vi "LSMcontroller_v59_PIzstage.vi"() -> ()   [LabVIEW 2015] (continued)
                n3606 = Unbundle By Name(w327) -> ("AOtab"=w308:dbl, "Repeats"=w326:dbl, "Cycles"=w325:dbl, "Start amplitude (V)"=w324:dbl, "Baseline (V)"=w323:dbl, "Step size (V)"=w322:dbl, "DC (%)"=w321:dbl, "Sampling frequency (Hz)"=w320:dbl, "Period (ms)"=w319:dbl, "Offset (V)"=w318:dbl, "Amplitude (V)"=w317:dbl, "Frequency"=w316:dbl, "Tri Repeats"=w315:dbl, "phase shift (ms)"=w314:dbl, "Pulses"=w313:dbl, "Tri phase"=w309:dbl, "padding value"=w305:dbl, "Matlab wave file"=w306:path)
                n3607 = To Unsigned Long Integer(number=w308) -> (unsigned 32bit integer=w307:u32)
                n3608 = local write "Build analog waveform tabs"(w307) -> ()
                n3609 = local write "Matlab waveform path"(w306) -> ()
                n3610 = local write "phase shift (ms)"(w314) -> ()
                n3611 = local write "Repeats"(w326) -> ()
                n3612 = local write "Cycles"(w325) -> ()
                n3613 = local write "Amplitude (V)"(w317) -> ()
                n3614 = local write "Matlab padding value"(w305) -> ()
                n3615 = local write "Tri padding value"(w305) -> ()
                n3616 = local write "Start amplitude (V)"(w324) -> ()
                n3617 = local write "Tri Phase (s)"(w309) -> ()
                n3618 = local write "Period (ms)"(w319) -> ()
                n3619 = local write "Tri Repeats"(w315) -> ()
                n3620 = local write "Offset (V)"(w318) -> ()
                n3621 = local write "Frequency"(w316) -> ()
                n3622 = local write "Pulses"(w313) -> ()
                n3623 = local write "padding value"(w305) -> ()
                n3624 = local write "Sampling rate \ncurrent wf"(w320) -> ()
                n3625 = local write "Baseline (V)"(w323) -> ()
                n3626 = local write "Step size (V)"(w322) -> ()
                n3627 = local write "DC (%)"(w321) -> ()
              }
              frame True {
              }
            }
          }
          event "Rem AO wave": Value Change {
            n3628 = event-data() -> ("NewVal"=w328:bool)  [unwired: 1 in, 5 out]
            n3629 = case shown="True" w328 {
              frame False {
              }
              frame True {
                n3630 = stacked-sequence {
                  seq-local: [_ _ w434 _ _ _ _] -> [_ _ _ _ w454 w457 _]
                  frame #0 {
                    n3631 = local read "Measurement"() -> (w329:T4)
                    n3632 = case shown="\"X-Y-t movie\", Default" w329 {
                      frame "X-Y-t movie", Default {
                        n3633 = local read "avpp"() -> (w350:i32)
                        n3634 = local read "Angle ref"() -> (w349:dbl)
                        n3635 = local read "ROI Type"() -> (w348:u16)
                        n3636 = local read "xpixels ref"() -> (w345:i32)
                        n3637 = local read "Vx-min ref"() -> (w344:dbl)
                        n3638 = local read "Vx-max ref"() -> (w343:dbl)
                        n3639 = local read "ypixels ref"() -> (w341:i32)
                        n3640 = local read "Vy-min ref"() -> (w342:dbl)
                        n3641 = local read "Vy-max ref"() -> (w338:dbl)
                        n3642 = local read "Sampling rate"() -> (w332:dbl)
                        n3643 = local read "finite samples"() -> (w333:bool)
                        n3644 = local read "continuous"() -> (w336:bool)
                        n3645 = local read "wavdet"() -> (w337:bool)
                        n3646 = local read "# of frames"() -> (w335:i32)
                        n3647 = local read "maxbufferAI"() -> (w334:i32)
                        n3648 = local read "Override AI buffer"() -> (w330:bool)
                        n3649 = call "2pparameters.vi"("command"="get") -> ("params out"=w347:T11)  [unwired: 1 in]
                        n3650 = Bundle By Name(cluster=w347, "type"="X-Y-t movie", "avpp"=w350, "Angle Img"=w349, "Xpixels Img"=w345, "Vx-min Img"=w344, "VX-max Img"=w343, "Ypixels Img"=w341, "Vy-min Img"=w342, "Vy-max Img"=w338, "srate"=w332, "srate Img"=w332, "finite"=w333, "cont"=w336, "wavdet"=w337, "measpoints"=w335, "maxbufferAI"=w334, "Drawing Mode"=w348, "Vz-reset"=0.0, "AIoverride"=w330) -> (w339:T11)
                        n3651 = call "2pparameters.vi"("Params in"=w339, "command"="set") -> ()  [unwired: 1 out]
                      }
                      frame "X-Y-Z stack" {
                        n3652 = call "2pparameters.vi"("command"="get") -> ("params out"=w354:T11)  [unwired: 1 in]
                        n3653 = Bundle By Name(cluster=w354, "type"="X-Y-Z stack") -> (w352:T11)
                        n3654 = call "2pparameters.vi"("Params in"=w352, "command"="set") -> ()  [unwired: 1 out]
                      }
                      frame "Lifetime (scan)" {
                        n3655 = call "2pparameters.vi"("command"="get") -> ("params out"=w359:T11)  [unwired: 1 in]
                        n3656 = Bundle By Name(cluster=w359, "type"="Lifetime (scan)") -> (w357:T11)
                        n3657 = call "2pparameters.vi"("Params in"=w357, "command"="set") -> ()  [unwired: 1 out]
                      }
                      frame "Lifetime (contour)" {
                        n3658 = local read "Vy-min draw"() -> (w369:dbl)
                        n3659 = local read "Vy-max draw"() -> (w368:dbl)
                        n3660 = local read "Vx-min draw"() -> (w371:dbl)
                        n3661 = local read "Vx-max draw"() -> (w370:dbl)
                        n3662 = local read "xpixels ref"() -> (w367:i32)
                        n3663 = local read "ypixels ref"() -> (w366:i32)
                        n3664 = local read "ROI Type"() -> (w365:u16)
                        n3665 = local read "srateAODOtt"() -> (w376:dbl)
                        n3666 = local read "# of frames"() -> (w381:i32)
                        n3667 = local read "refreshtime"() -> (w373:dbl)
                        n3668 = local read "Pel"() -> (w364:dbl)
                        n3669 = local read "bin"() -> (w379:dbl)
                        n3670 = local read "Override AI buffer"() -> (w362:bool)
                        n3671 = local read "finite samples"() -> (w388:bool)
                        n3672 = local read "srateAODOtt"() -> (w375:dbl)
                        n3673 = local read "srateAODOtt"() -> (w382:dbl)
                        n3674 = local read "continuous"() -> (w387:bool)
                        n3675 = local read "Angle ref"() -> (w372:dbl)
                        n3676 = local read "wavdet"() -> (w389:bool)
                        n3677 = local read "Vx-ref"() -> (w384:dbl)
                        n3678 = local read "Vy-ref"() -> (w386:dbl)
                        n3679 = local read "avpp"() -> (w385:i32)
                        n3680 = call "tt_timeandsamples.vi"("bin"=w379, "refreshtime"=w373, "srateAODOtt"=w376, "tot#ofsamples"=w381) -> ("refreshrate"=w377:dbl, "refreshbuffer"=w378:i32, "timetracecycles"=w383:i32)  [unwired: 5 in]
                        n3681 = local read "bin"() -> (w380:dbl)
                        n3682 = call "2pparameters.vi"("command"="get") -> ("params out"=w392:T11)  [unwired: 1 in]
                        n3683 = Bundle By Name(cluster=w392, "Drawing Mode"=w365, "measpoints"=w381, "tt_cycles"=w383, "refreshbuffer"=w378, "refreshrate"=w377, "Vx-ref"=w384, "Vy-ref"=w386, "srate"=w375, "finite"=w388, "cont"=w387, "wavdet"=w389, "avpp"=w385, "srateAODO"=w382, "bufferAI"=w378, "bin"=w380, "Angle Img"=w372, "Vxminref"=w371, "Vxmaxref"=w370, "Vyminref"=w369, "Vymaxref"=w368, "Xpixels Img"=w367, "Ypixels Img"=w366, "Pel"=w364, "Vz-reset"=0.0, "AIoverride"=w362, "type"="Lifetime (contour)") -> (w390:T11)
                        n3684 = Reciprocal(x=w377) -> (1/x=w374:dbl)
                        n3685 = local write "refreshtime"(w374) -> ()
                        n3686 = call "2pparameters.vi"("Params in"=w390, "command"="set") -> ()  [unwired: 1 out]
                      }
                      frame "X-Y-Z-t movie" {
                      }
                      frame "linescan" {
                      }
                      frame "Timetrace" {
                        n3687 = local read "Vy-min draw"() -> (w402:dbl)
                        n3688 = local read "Vy-max draw"() -> (w401:dbl)
                        n3689 = local read "Vx-min draw"() -> (w404:dbl)
                        n3690 = local read "Vx-max draw"() -> (w403:dbl)
                        n3691 = local read "xpixels ref"() -> (w400:i32)
                        n3692 = local read "ypixels ref"() -> (w399:i32)
                        n3693 = local read "ROI Type"() -> (w398:u16)
                        n3694 = local read "srateAODOtt"() -> (w409:dbl)
                        n3695 = local read "# of frames"() -> (w414:i32)
                        n3696 = local read "refreshtime"() -> (w406:dbl)
                        n3697 = local read "Pel"() -> (w397:dbl)
                        n3698 = local read "bin"() -> (w412:dbl)
                        n3699 = local read "Override AI buffer"() -> (w395:bool)
                        n3700 = local read "finite samples"() -> (w421:bool)
                        n3701 = local read "srateAODOtt"() -> (w408:dbl)
                        n3702 = local read "srateAODOtt"() -> (w415:dbl)
                        n3703 = local read "continuous"() -> (w420:bool)
                        n3704 = local read "Angle ref"() -> (w405:dbl)
                        n3705 = local read "wavdet"() -> (w422:bool)
                        n3706 = local read "Vx-ref"() -> (w417:dbl)
                        n3707 = local read "Vy-ref"() -> (w419:dbl)
                        n3708 = local read "avpp"() -> (w418:i32)
                        n3709 = call "tt_timeandsamples.vi"("bin"=w412, "refreshtime"=w406, "srateAODOtt"=w409, "tot#ofsamples"=w414) -> ("refreshrate"=w410:dbl, "refreshbuffer"=w411:i32, "timetracecycles"=w416:i32)  [unwired: 5 in]
                        n3710 = local read "bin"() -> (w413:dbl)
                        n3711 = call "2pparameters.vi"("command"="get") -> ("params out"=w425:T11)  [unwired: 1 in]
                        n3712 = Bundle By Name(cluster=w425, "Drawing Mode"=w398, "measpoints"=w414, "tt_cycles"=w416, "refreshbuffer"=w411, "refreshrate"=w410, "Vx-ref"=w417, "Vy-ref"=w419, "srate"=w408, "finite"=w421, "cont"=w420, "wavdet"=w422, "avpp"=w418, "srateAODO"=w415, "bufferAI"=w411, "bin"=w413, "Angle Img"=w405, "Vxminref"=w404, "Vxmaxref"=w403, "Vyminref"=w402, "Vymaxref"=w401, "Xpixels Img"=w400, "Ypixels Img"=w399, "Pel"=w397, "Vz-reset"=0.0, "AIoverride"=w395, "type"="Timetrace") -> (w423:T11)
                        n3713 = Reciprocal(x=w410) -> (1/x=w407:dbl)
                        n3714 = local write "refreshtime"(w407) -> ()
                        n3715 = call "2pparameters.vi"("Params in"=w423, "command"="set") -> ()  [unwired: 1 out]
                      }
                      frame "Lifetime (point)" {
                      }
                    }
                  }
                  frame #1 {
                    w428 = FALSE ("wavdet")
                    n3716 = call "2pparameters.vi"("command"="get") -> ("params out"=w432:T11)  [unwired: 1 in]
                    n3717 = Bundle By Name(cluster=w432, "finite"=w428, "cont"=w428, "wavdet"=TRUE) -> (w429:T11)
                    n3718 = call "2pparameters.vi"("Params in"=w429, "command"="set") -> ()  [unwired: 1 out]
                  }
                  frame #2 {
                    # "remove channel from numbers array"
                    n3719 = local read "AO channels"() -> (w439:u32)
                    n3720 = call "2pparameters.vi"("command"="get") -> ("params out"=w437:T11)  [unwired: 1 in]
                    n3721 = in-place {
                      in-place-border: w439 -> [w445]
                      in-place-border: [w442] -> w440
                      in-place-border: [w441] -> w434
                      n3722 = in-place-cluster #50(w437) -> ("aAO"=w444:u32[])
                      n3723 = call "remove channel from active arrayv2.vi"("line array in"=w444, "line to remove"=w445) -> ("line array out"=w443:u32[], "removal"=w442:bool, "index"=w441:i32)
                      n3724 = in-place-cluster #50("aAO"=w443) -> (w435:T11)
                    }
                    n3725 = local write "remAO"(w440) -> ()
                    n3726 = call "2pparameters.vi"("Params in"=w435, "command"="set") -> ()  [unwired: 1 out]
                  }
                  frame #3 {
                    n3727 = local read "remAO"() -> (w446:bool)
                    n3728 = case shown="True" w446 {
                      frame False {
                      }
                      frame True {
                        n3729 = call "Used AO lines.vi"() -> ("used AO names"=w450:string[], "used AO lines"=w452:tag[])  [unwired: 2 in]
                        n3730 = control-ref of="Analog Lines Plot"() -> (w451:refnum<vi>)
                        n3731 = control-ref of="Digital Lines Plot"() -> (w449:refnum<vi>)
                        n3732 = call "Used DO lines.vi"() -> ("used DO names"=w448:string[], "used DO lines"=w447:tag[])  [unwired: 2 in]
                        n3733 = local write "Analog Used Lines"(w452) -> ()
                        n3734 = local write "Analog Used Names"(w450) -> ()
                        n3735 = local write "Digital Used Lines"(w447) -> ()
                        n3736 = local write "Digital Used Names"(w448) -> ()
                        n3737 = call "prepDOWaveplot.vi"("DigitalGraph in"=w449, "used DO names"=w448) -> ()  [unwired: 1 in]
                        n3738 = call "prepAOWaveplot.vi"("WaveformGraph in"=w451, "Analog Used Names"=w450) -> ()  [unwired: 1 in]
                      }
                    }
                  }
                  frame #4 {
                    n3739 = local read "remAO"() -> (w453:bool)
                    n3740 = case shown="True" w453 {
                      tunnel: w454 -> [_ w455]
                      frame False {
                      }
                      frame True {
                        n3741 = call "waveformparamsv2.vi"("command"="rem AO", "index"=w455) -> ()  [unwired: 3 in, 3 out]
                      }
                    }
                  }
                  frame #5 {
                    n3742 = local read "remAO"() -> (w458:bool)
                    n3743 = case shown="True" w458 {
                      tunnel: w457 -> [_ w477]
                      frame False {
                      }
                      frame True {
                        n3744 = local read "Meastab"() -> (w462:enum32{"X-Y Image", "Linescan", "Timetrace"})
                        n3745 = property on="refwf" class="Ring (strict)"() -> ("RingText.Text"=w465:string)  [unwired: 2 in, 2 out]
                        n3746 = case shown="\"Timetrace\"" w462 {
                          tunnel: [w478 w479] -> w461
                          frame "X-Y Image", Default {
                            n3747 = local read "Sampling rate"() -> (w478:dbl)
                          }
                          frame "Timetrace" {
                            n3748 = local read "srateAODOtt"() -> (w479:dbl)
                          }
                        }
                        n3749 = call "waveformsAObuffer.vi"("command"="get") -> ("AO wf out"=w474:waveform(dbl)[])  [unwired: 1 in]
                        n3750 = call "waveformsDObuffer.vi"("command"="get") -> ("DO wf out"=w471:digitalwaveform[])  [unwired: 1 in]
                        n3751 = Delete From Array(array=w474, length=1, index=w477) -> (array with subset deleted=w466:waveform(dbl)[])  [unwired: 1 out]
                        n3752 = call "correctwaveformsizetemp.vi"("new sampling frequency (Hz)"=w461, "start"=FALSE, "reference waveforms to"=w465, "Analog waveforms in"=w466, "stop"=FALSE, "Digital waveforms in"=w471) -> ("analog wf out"=w469:waveform(dbl)[], "Digital wf out"=w467:digitalwaveform[], "measpoints"=w463:i32)
                        n3753 = local write "Analog Lines Plot"(w469) -> ()
                        n3754 = call "GetNumCamFramesv2.vi"("Digital Waveform Graph"=w467) -> ("Numeric"=w468:i32)  [unwired: 10 in]
                        n3755 = local write "Digital Lines Plot"(w467) -> ()
                        n3756 = call "waveformsAObuffer.vi"("AO wf in"=w469, "command"="set") -> ()  [unwired: 1 out]
                        n3757 = call "waveformsDObuffer.vi"("DO wf in"=w467, "command"="set") -> ()  [unwired: 1 out]
                        n3758 = local read "wavdet"() -> (w464:bool)
                        n3759 = local write "Total Camera Frames"(w468) -> ()
                        n3760 = case shown="True" w464 {
                          tunnel: w463 -> [_ w480]
                          frame False {
                          }
                          frame True {
                            n3761 = local write "# of frames"(w480) -> ()
                          }
                        }
                      }
                    }
                  }
                  frame #6 {
                    w481 = FALSE ("remAO")
                    n3762 = local read "finite samples"() -> (w482:bool)
                    n3763 = local read "continuous"() -> (w483:bool)
                    n3764 = local read "wavdet"() -> (w484:bool)
                    n3765 = call "2pparameters.vi"("command"="get") -> ("params out"=w487:T11)  [unwired: 1 in]
                    n3766 = Bundle By Name(cluster=w487, "finite"=w482, "cont"=w483, "wavdet"=w484) -> (w485:T11)
                    n3767 = local write "remAO"(w481) -> ()
                    n3768 = property on="Rem AO wave" class="Bool (strict)"("Val(Sgnl)"=w481) -> ()  [unwired: 2 in, 2 out]
                    n3769 = call "2pparameters.vi"("Params in"=w485, "command"="set") -> ()  [unwired: 1 out]
                  }
                }
              }
            }
          }
          event "Add DO wave": Value Change {
            n3770 = event-data() -> ("NewVal"=w489:bool)  [unwired: 1 in, 5 out]
            n3771 = case shown="True" w489 {
              frame False {
              }
              frame True {
                n3772 = stacked-sequence {
                  seq-local: [_ _ _ _ _ w649 _ _] -> [_ _ _ _ _ _ w664 _]
                  frame #0 {
                    n3773 = local read "Measurement"() -> (w490:T4)
                    n3774 = case shown="\"X-Y-t movie\", Default" w490 {
                      frame "X-Y-t movie", Default {
                        n3775 = local read "avpp"() -> (w511:i32)
                        n3776 = local read "Angle ref"() -> (w510:dbl)
                        n3777 = local read "ROI Type"() -> (w509:u16)
                        n3778 = local read "xpixels ref"() -> (w506:i32)
                        n3779 = local read "Vx-min ref"() -> (w505:dbl)
                        n3780 = local read "Vx-max ref"() -> (w504:dbl)
                        n3781 = local read "ypixels ref"() -> (w502:i32)
                        n3782 = local read "Vy-min ref"() -> (w503:dbl)
                        n3783 = local read "Vy-max ref"() -> (w499:dbl)
                        n3784 = local read "Sampling rate"() -> (w493:dbl)
                        n3785 = local read "finite samples"() -> (w494:bool)
                        n3786 = local read "continuous"() -> (w497:bool)
                        n3787 = local read "wavdet"() -> (w498:bool)
                        n3788 = local read "# of frames"() -> (w496:i32)
                        n3789 = local read "maxbufferAI"() -> (w495:i32)
                        n3790 = local read "Override AI buffer"() -> (w491:bool)
                        n3791 = call "2pparameters.vi"("command"="get") -> ("params out"=w508:T11)  [unwired: 1 in]
                        n3792 = Bundle By Name(cluster=w508, "type"="X-Y-t movie", "avpp"=w511, "Angle Img"=w510, "Xpixels Img"=w506, "Vx-min Img"=w505, "VX-max Img"=w504, "Ypixels Img"=w502, "Vy-min Img"=w503, "Vy-max Img"=w499, "srate"=w493, "srate Img"=w493, "finite"=w494, "cont"=w497, "wavdet"=w498, "measpoints"=w496, "maxbufferAI"=w495, "Drawing Mode"=w509, "Vz-reset"=0.0, "AIoverride"=w491) -> (w500:T11)
                        n3793 = call "2pparameters.vi"("Params in"=w500, "command"="set") -> ()  [unwired: 1 out]
                      }
                      frame "X-Y-Z stack" {
                        n3794 = call "2pparameters.vi"("command"="get") -> ("params out"=w515:T11)  [unwired: 1 in]
                        n3795 = Bundle By Name(cluster=w515, "type"="X-Y-Z stack") -> (w513:T11)
                        n3796 = call "2pparameters.vi"("Params in"=w513, "command"="set") -> ()  [unwired: 1 out]
                      }
                      frame "Lifetime (scan)" {
                        n3797 = call "2pparameters.vi"("command"="get") -> ("params out"=w520:T11)  [unwired: 1 in]
                        n3798 = Bundle By Name(cluster=w520, "type"="Lifetime (scan)") -> (w518:T11)
                        n3799 = call "2pparameters.vi"("Params in"=w518, "command"="set") -> ()  [unwired: 1 out]
                      }
                      frame "Lifetime (contour)" {
                        n3800 = local read "Vy-min draw"() -> (w530:dbl)
                        n3801 = local read "Vy-max draw"() -> (w529:dbl)
                        n3802 = local read "Vx-min draw"() -> (w532:dbl)
                        n3803 = local read "Vx-max draw"() -> (w531:dbl)
                        n3804 = local read "xpixels ref"() -> (w528:i32)
                        n3805 = local read "ypixels ref"() -> (w527:i32)
                        n3806 = local read "ROI Type"() -> (w526:u16)
                        n3807 = local read "srateAODOtt"() -> (w537:dbl)
                        n3808 = local read "# of frames"() -> (w542:i32)
                        n3809 = local read "refreshtime"() -> (w534:dbl)
                        n3810 = local read "Pel"() -> (w525:dbl)
                        n3811 = local read "bin"() -> (w540:dbl)
                        n3812 = local read "Override AI buffer"() -> (w523:bool)
                        n3813 = local read "finite samples"() -> (w549:bool)
                        n3814 = local read "srateAODOtt"() -> (w536:dbl)
                        n3815 = local read "srateAODOtt"() -> (w543:dbl)
                        n3816 = local read "continuous"() -> (w548:bool)
                        n3817 = local read "Angle ref"() -> (w533:dbl)
                        n3818 = local read "wavdet"() -> (w550:bool)
                        n3819 = local read "Vx-ref"() -> (w545:dbl)
                        n3820 = local read "Vy-ref"() -> (w547:dbl)
                        n3821 = local read "avpp"() -> (w546:i32)
                        n3822 = call "tt_timeandsamples.vi"("bin"=w540, "refreshtime"=w534, "srateAODOtt"=w537, "tot#ofsamples"=w542) -> ("refreshrate"=w538:dbl, "refreshbuffer"=w539:i32, "timetracecycles"=w544:i32)  [unwired: 5 in]
                        n3823 = local read "bin"() -> (w541:dbl)
                        n3824 = call "2pparameters.vi"("command"="get") -> ("params out"=w553:T11)  [unwired: 1 in]
                        n3825 = Bundle By Name(cluster=w553, "Drawing Mode"=w526, "measpoints"=w542, "tt_cycles"=w544, "refreshbuffer"=w539, "refreshrate"=w538, "Vx-ref"=w545, "Vy-ref"=w547, "srate"=w536, "finite"=w549, "cont"=w548, "wavdet"=w550, "avpp"=w546, "srateAODO"=w543, "bufferAI"=w539, "bin"=w541, "Angle Img"=w533, "Vxminref"=w532, "Vxmaxref"=w531, "Vyminref"=w530, "Vymaxref"=w529, "Xpixels Img"=w528, "Ypixels Img"=w527, "Pel"=w525, "Vz-reset"=0.0, "AIoverride"=w523, "type"="Lifetime (contour)") -> (w551:T11)
                        n3826 = Reciprocal(x=w538) -> (1/x=w535:dbl)
                        n3827 = local write "refreshtime"(w535) -> ()
                        n3828 = call "2pparameters.vi"("Params in"=w551, "command"="set") -> ()  [unwired: 1 out]
                      }
                      frame "X-Y-Z-t movie" {
                      }
                      frame "linescan" {
                      }
                      frame "Timetrace" {
                        n3829 = local read "Vy-min draw"() -> (w563:dbl)
                        n3830 = local read "Vy-max draw"() -> (w562:dbl)
                        n3831 = local read "Vx-min draw"() -> (w565:dbl)
                        n3832 = local read "Vx-max draw"() -> (w564:dbl)
                        n3833 = local read "xpixels ref"() -> (w561:i32)
                        n3834 = local read "ypixels ref"() -> (w560:i32)
                        n3835 = local read "ROI Type"() -> (w559:u16)
                        n3836 = local read "srateAODOtt"() -> (w570:dbl)
                        n3837 = local read "# of frames"() -> (w575:i32)
                        n3838 = local read "refreshtime"() -> (w567:dbl)
                        n3839 = local read "Pel"() -> (w558:dbl)
                        n3840 = local read "bin"() -> (w573:dbl)
                        n3841 = local read "Override AI buffer"() -> (w556:bool)
                        n3842 = local read "finite samples"() -> (w582:bool)
                        n3843 = local read "srateAODOtt"() -> (w569:dbl)
                        n3844 = local read "srateAODOtt"() -> (w576:dbl)
                        n3845 = local read "continuous"() -> (w581:bool)
                        n3846 = local read "Angle ref"() -> (w566:dbl)
                        n3847 = local read "wavdet"() -> (w583:bool)
                        n3848 = local read "Vx-ref"() -> (w578:dbl)
                        n3849 = local read "Vy-ref"() -> (w580:dbl)
                        n3850 = local read "avpp"() -> (w579:i32)
                        n3851 = call "tt_timeandsamples.vi"("bin"=w573, "refreshtime"=w567, "srateAODOtt"=w570, "tot#ofsamples"=w575) -> ("refreshrate"=w571:dbl, "refreshbuffer"=w572:i32, "timetracecycles"=w577:i32)  [unwired: 5 in]
                        n3852 = local read "bin"() -> (w574:dbl)
                        n3853 = call "2pparameters.vi"("command"="get") -> ("params out"=w586:T11)  [unwired: 1 in]
                        n3854 = Bundle By Name(cluster=w586, "Drawing Mode"=w559, "measpoints"=w575, "tt_cycles"=w577, "refreshbuffer"=w572, "refreshrate"=w571, "Vx-ref"=w578, "Vy-ref"=w580, "srate"=w569, "finite"=w582, "cont"=w581, "wavdet"=w583, "avpp"=w579, "srateAODO"=w576, "bufferAI"=w572, "bin"=w574, "Angle Img"=w566, "Vxminref"=w565, "Vxmaxref"=w564, "Vyminref"=w563, "Vymaxref"=w562, "Xpixels Img"=w561, "Ypixels Img"=w560, "Pel"=w558, "Vz-reset"=0.0, "AIoverride"=w556, "type"="Timetrace") -> (w584:T11)
                        n3855 = Reciprocal(x=w571) -> (1/x=w568:dbl)
                        n3856 = local write "refreshtime"(w568) -> ()
                        n3857 = call "2pparameters.vi"("Params in"=w584, "command"="set") -> ()  [unwired: 1 out]
                      }
                      frame "Lifetime (point)" {
                      }
                    }
                  }
                  frame #1 {
                    w589 = FALSE ("wavdet")
                    n3858 = call "2pparameters.vi"("command"="get") -> ("params out"=w593:T11)  [unwired: 1 in]
                    n3859 = Bundle By Name(cluster=w593, "finite"=w589, "cont"=w589, "wavdet"=TRUE) -> (w590:T11)
                    n3860 = call "2pparameters.vi"("Params in"=w590, "command"="set") -> ()  [unwired: 1 out]
                  }
                  frame #2 {
                    n3861 = local read "DO channels"() -> (w600:u16)
                    n3862 = call "2pparameters.vi"("command"="get") -> ("params out"=w598:T11)  [unwired: 1 in]
                    n3863 = in-place {
                      in-place-border: w600 -> [w604]
                      in-place-border: [w601] -> w595
                      n3864 = in-place-cluster #51(w598) -> ("aDO"=w603:u32[])
                      n3865 = call "add channel to active arrayv2.vi"("line array in"=w603, "line to add"=w604) -> ("line array out"=w602:u32[], "addition"=w601:bool)  [unwired: 1 out]
                      n3866 = in-place-cluster #51("aDO"=w602) -> (w596:T11)
                    }
                    n3867 = local write "addDO"(w595) -> ()
                    n3868 = call "2pparameters.vi"("Params in"=w596, "command"="set") -> ()  [unwired: 1 out]
                  }
                  frame #3 {
                    n3869 = local read "addDO"() -> (w605:bool)
                    n3870 = case shown="True" w605 {
                      frame False {
                      }
                      frame True {
                        n3871 = call "Used AO lines.vi"() -> ("used AO names"=w609:string[], "used AO lines"=w611:tag[])  [unwired: 2 in]
                        n3872 = control-ref of="Analog Lines Plot"() -> (w610:refnum<vi>)
                        n3873 = control-ref of="Digital Lines Plot"() -> (w608:refnum<vi>)
                        n3874 = call "Used DO lines.vi"() -> ("used DO names"=w607:string[], "used DO lines"=w606:tag[])  [unwired: 2 in]
                        n3875 = local write "Analog Used Lines"(w611) -> ()
                        n3876 = local write "Analog Used Names"(w609) -> ()
                        n3877 = local write "Digital Used Lines"(w606) -> ()
                        n3878 = local write "Digital Used Names"(w607) -> ()
                        n3879 = call "prepDOWaveplot.vi"("DigitalGraph in"=w608, "used DO names"=w607) -> ()  [unwired: 1 in]
                        n3880 = call "prepAOWaveplot.vi"("WaveformGraph in"=w610, "Analog Used Names"=w609) -> ()  [unwired: 1 in]
                      }
                    }
                  }
                  frame #4 {
                    n3881 = local read "addDO"() -> (w612:bool)
                    n3882 = case shown="True" w612 {
                      frame False {
                      }
                      frame True {
                        n3883 = local read "Build digital waveform tabs"() -> (w613:enum32{"Simple", "Matlab"})
                        n3884 = case shown="\"Matlab\"" w613 {
                          frame "Simple", Default {
                            n3885 = local read "Meastab"() -> (w615:enum32{"X-Y Image", "Linescan", "Timetrace"})
                            n3886 = call "waveformparamsv2.vi"("command"="get") -> ("Params out"=w629:T15)  [unwired: 4 in, 2 out]
                            n3887 = case shown="\"Timetrace\"" w615 {
                              tunnel: [w631 w632] -> w614
                              frame "X-Y Image", Default {
                                n3888 = local read "Sampling rate"() -> (w631:dbl)
                              }
                              frame "Timetrace" {
                                n3889 = local read "srateAODOtt"() -> (w632:dbl)
                              }
                            }
                            n3890 = Unbundle By Name(w629) -> ("DO parameters"=w627:T18)
                            n3891 = local read "Digital padding value"() -> (w618:dbl)
                            n3892 = local read "Digital time offset (s)"() -> (w619:dbl)
                            n3893 = local read "Digital phase (s)"() -> (w621:dbl)
                            n3894 = local read "Digital Freq (Hz)"() -> (w620:dbl)
                            n3895 = local read "Digital DC (%)"() -> (w622:dbl)
                            n3896 = Index Array(array=w627, index=0) -> (element=w626:T19)
                            n3897 = Bundle By Name(cluster=w626, "Digital DC (%)"=w622, "Digital phase"=w621, "Digital Freq (Hz)"=w620, "Sampling frequency (Hz)"=w614, "Digital time offset (s)"=w619, "padding value"=w618, "matlab wave file"=path "", "DOtab"=0.0) -> (w624:T19)
                            n3898 = Build Array(w624) -> (w623:T18)
                            n3899 = call "waveformparamsv2.vi"("command"="add DO", "add DO"=w623) -> ()  [unwired: 3 in, 3 out]
                          }
                          frame "Matlab" {
                            w636 = 0.0 ("DOtab")
                            n3900 = local read "Meastab"() -> (w634:enum32{"X-Y Image", "Linescan", "Timetrace"})
                            n3901 = call "waveformparamsv2.vi"("command"="get") -> ("Params out"=w645:T15)  [unwired: 4 in, 2 out]
                            n3902 = case shown="\"Timetrace\"" w634 {
                              tunnel: [w647 w648] -> w633
                              frame "X-Y Image", Default {
                                n3903 = local read "Sampling rate"() -> (w647:dbl)
                              }
                              frame "Timetrace" {
                                n3904 = local read "srateAODOtt"() -> (w648:dbl)
                              }
                            }
                            n3905 = Unbundle By Name(w645) -> ("DO parameters"=w643:T18)
                            n3906 = local read "Matlab waveform path DO"() -> (w635:path)
                            n3907 = local read "Matlab padding value DO"() -> (w638:dbl)
                            n3908 = Index Array(array=w643, index=0) -> (element=w642:T19)
                            n3909 = Bundle By Name(cluster=w642, "Digital DC (%)"=w636, "Digital phase"=w636, "Digital Freq (Hz)"=w636, "Sampling frequency (Hz)"=w633, "Digital time offset (s)"=w636, "padding value"=w638, "matlab wave file"=w635, "DOtab"=1.0) -> (w640:T19)
                            n3910 = Build Array(w640) -> (w639:T18)
                            n3911 = call "waveformparamsv2.vi"("command"="add DO", "add DO"=w639) -> ()  [unwired: 3 in, 3 out]
                          }
                        }
                      }
                    }
                  }
                  frame #5 {
                    n3912 = local read "addDO"() -> (w650:bool)
                    n3913 = case shown="True" w650 {
                      tunnel: [_ w651] -> w649
                      frame False {
                      }
                      frame True {
                        n3914 = property on="refwf" class="Ring (strict)"() -> ("RingText.Text"=w656:string)  [unwired: 2 in, 2 out]
                        n3915 = call "waveformsDObuffer.vi"("command"="get") -> ("DO wf out"=w655:digitalwaveform[])  [unwired: 1 in]
                        n3916 = call "waveformsAObuffer.vi"("command"="get") -> ("AO wf out"=w653:waveform(dbl)[])  [unwired: 1 in]
                        n3917 = call "referfencesize.vi"("Digital waveforms in"=w655, "Analog waveforms in"=w653, "reference waveforms to"=w656) -> ("number of samples"=w651:i32)  [unwired: 2 in]
                      }
                    }
                  }
                  frame #6 {
                    n3918 = local read "Build digital waveform tabs"() -> (w667:enum32{"Simple", "Matlab"})
                    n3919 = call "waveformparamsv2.vi"("command"="get last DO") -> ("last DO"=w666:T19)  [unwired: 4 in, 2 out]
                    n3920 = local read "Meastab"() -> (w660:enum32{"X-Y Image", "Linescan", "Timetrace"})
                    n3921 = call "waveformsDObuffer.vi"("command"="get") -> ("DO wf out"=w665:digitalwaveform[])  [unwired: 1 in]
                    n3922 = case shown="\"Simple\", Default" w667 {
                      tunnel: w666 -> [w684 w686]
                      tunnel: w664 -> [w683 _]
                      tunnel: [w682 w685] -> w663
                      frame "Simple", Default {
                        n3923 = call "simple digital from wf params.vi"("waveform params"=w684, "number of samples"=w683) -> ("digital waveform"=w682:digitalwaveform)
                      }
                      frame "Matlab" {
                        n3924 = call "matlabDOwffromparam.vi"("waveform params"=w686) -> ("digital waveform"=w685:digitalwaveform)
                      }
                    }
                    n3925 = property on="refwf" class="Ring (strict)"() -> ("RingText.Text"=w670:string)  [unwired: 2 in, 2 out]
                    n3926 = case shown="\"Timetrace\"" w660 {
                      tunnel: [w679 w680] -> w659
                      frame "X-Y Image", Default {
                        n3927 = local read "Sampling rate"() -> (w679:dbl)
                      }
                      frame "Timetrace" {
                        n3928 = local read "srateAODOtt"() -> (w680:dbl)
                      }
                    }
                    n3929 = call "waveformsAObuffer.vi"("command"="get") -> ("AO wf out"=w678:waveform(dbl)[])  [unwired: 1 in]
                    n3930 = Build Array (concatenate)(w665, w663) -> (w669:digitalwaveform[])
                    n3931 = call "correctwaveformsizetemp.vi"("new sampling frequency (Hz)"=w659, "start"=FALSE, "reference waveforms to"=w670, "Analog waveforms in"=w678, "stop"=FALSE, "Digital waveforms in"=w669) -> ("analog wf out"=w673:waveform(dbl)[], "Digital wf out"=w671:digitalwaveform[], "measpoints"=w661:i32)
                    n3932 = local write "Analog Lines Plot"(w673) -> ()
                    n3933 = call "GetNumCamFramesv2.vi"("Digital Waveform Graph"=w671) -> ("Numeric"=w672:i32)  [unwired: 10 in]
                    n3934 = local write "Digital Lines Plot"(w671) -> ()
                    n3935 = call "waveformsAObuffer.vi"("AO wf in"=w673, "command"="set") -> ()  [unwired: 1 out]
                    n3936 = call "waveformsDObuffer.vi"("DO wf in"=w671, "command"="set") -> ()  [unwired: 1 out]
                    n3937 = local write "Total Camera Frames"(w672) -> ()
                    n3938 = local read "wavdet"() -> (w662:bool)
                    n3939 = case shown="True" w662 {
                      tunnel: w661 -> [_ w681]
                      frame False {
                      }
                      frame True {
                        n3940 = local write "# of frames"(w681) -> ()
                      }
                    }
                  }
                  frame #7 {
                    w687 = FALSE ("addAO")
                    n3941 = local read "finite samples"() -> (w688:bool)
                    n3942 = local read "continuous"() -> (w689:bool)
                    n3943 = local read "wavdet"() -> (w690:bool)
                    n3944 = call "2pparameters.vi"("command"="get") -> ("params out"=w693:T11)  [unwired: 1 in]
                    n3945 = Bundle By Name(cluster=w693, "finite"=w688, "cont"=w689, "wavdet"=w690) -> (w691:T11)
                    n3946 = call "2pparameters.vi"("Params in"=w691, "command"="set") -> ()  [unwired: 1 out]
                    n3947 = local write "addDO"(w687) -> ()
                    n3948 = property on="Add DO wave" class="Bool (strict)"("Val(Sgnl)"=w687) -> ()  [unwired: 2 in, 2 out]
                  }
                }
              }
            }
          }
          event "DO channels": Value Change {
            n3949 = event-data() -> ()  [unwired: 1 in, 6 out]
            n3950 = local read "DO channels"() -> (w697:u16)
            n3951 = call "2pparameters.vi"("command"="get") -> ("params out"=w699:T11)  [unwired: 1 in]
            n3952 = Unbundle By Name(w699) -> ("aDO"=w698:u32[])
            n3953 = Search 1D Array(1D array=w698, element=w697) -> (index of element=w696:i32)  [unwired: 1 in]
            n3954 = Equal?(x=w696, y=-1.0) -> (x = y?=w695:bool)
            n3955 = case shown="False" w695 {
              tunnel: w696 -> [w714 _]
              frame False {
                n3956 = call "waveformparamsv2.vi"("command"="get") -> ("Params out"=w709:T15)  [unwired: 4 in, 2 out]
                n3957 = Unbundle By Name(w709) -> ("DO parameters"=w707:T18)
                n3958 = Index Array(array=w707, index=w714) -> (element=w713:T19)
                n3959 = Unbundle By Name(w713) -> ("Digital DC (%)"=w712:dbl, "Digital phase"=w711:dbl, "Digital Freq (Hz)"=w710:dbl, "Sampling frequency (Hz)"=w702:dbl, "Digital time offset (s)"=w706:dbl, "padding value"=w705:dbl, "matlab wave file"=w704:path, "DOtab"=w703:dbl)
                n3960 = local write "Build digital waveform tabs"(w703) -> ()
                n3961 = local write "Digital DC (%)"(w712) -> ()
                n3962 = local write "Matlab waveform path DO"(w704) -> ()
                n3963 = local write "Digital time offset (s)"(w706) -> ()
                n3964 = local write "Matlab padding value DO"(w705) -> ()
                n3965 = local write "Digital padding value"(w705) -> ()
                n3966 = local write "Sampling rate \ncurrent wf"(w702) -> ()
                n3967 = local write "Digital Freq (Hz)"(w710) -> ()
                n3968 = local write "Digital phase (s)"(w711) -> ()
              }
              frame True {
              }
            }
          }
          event "Rem DO wave": Value Change {
            n3969 = event-data() -> ("NewVal"=w715:bool)  [unwired: 1 in, 5 out]
            n3970 = case shown="True" w715 {
              frame False {
              }
              frame True {
                n3971 = stacked-sequence {
                  seq-local: [_ _ w821 _ _ _ _] -> [_ _ _ _ w840 w851 _]
                  frame #0 {
                    n3972 = local read "Measurement"() -> (w716:T4)
                    n3973 = case shown="\"linescan\"" w716 {
                      frame "X-Y-t movie", Default {
                        n3974 = local read "avpp"() -> (w737:i32)
                        n3975 = local read "Angle ref"() -> (w736:dbl)
                        n3976 = local read "ROI Type"() -> (w735:u16)
                        n3977 = local read "xpixels ref"() -> (w732:i32)
                        n3978 = local read "Vx-min ref"() -> (w731:dbl)
                        n3979 = local read "Vx-max ref"() -> (w730:dbl)
                        n3980 = local read "ypixels ref"() -> (w728:i32)
                        n3981 = local read "Vy-min ref"() -> (w729:dbl)
                        n3982 = local read "Vy-max ref"() -> (w725:dbl)
                        n3983 = local read "Sampling rate"() -> (w719:dbl)
                        n3984 = local read "finite samples"() -> (w720:bool)
                        n3985 = local read "continuous"() -> (w723:bool)
                        n3986 = local read "wavdet"() -> (w724:bool)
                        n3987 = local read "# of frames"() -> (w722:i32)
                        n3988 = local read "maxbufferAI"() -> (w721:i32)
                        n3989 = local read "Override AI buffer"() -> (w717:bool)
                        n3990 = call "2pparameters.vi"("command"="get") -> ("params out"=w734:T11)  [unwired: 1 in]
                        n3991 = Bundle By Name(cluster=w734, "type"="X-Y-t movie", "avpp"=w737, "Angle Img"=w736, "Xpixels Img"=w732, "Vx-min Img"=w731, "VX-max Img"=w730, "Ypixels Img"=w728, "Vy-min Img"=w729, "Vy-max Img"=w725, "srate"=w719, "srate Img"=w719, "finite"=w720, "cont"=w723, "wavdet"=w724, "measpoints"=w722, "maxbufferAI"=w721, "Drawing Mode"=w735, "Vz-reset"=0.0, "AIoverride"=w717) -> (w726:T11)
                        n3992 = call "2pparameters.vi"("Params in"=w726, "command"="set") -> ()  [unwired: 1 out]
                      }
                      frame "X-Y-Z stack" {
                        n3993 = call "2pparameters.vi"("command"="get") -> ("params out"=w741:T11)  [unwired: 1 in]
                        n3994 = Bundle By Name(cluster=w741, "type"="X-Y-Z stack") -> (w739:T11)
                        n3995 = call "2pparameters.vi"("Params in"=w739, "command"="set") -> ()  [unwired: 1 out]
                      }
                      frame "Lifetime (scan)" {
                        n3996 = call "2pparameters.vi"("command"="get") -> ("params out"=w746:T11)  [unwired: 1 in]
                        n3997 = Bundle By Name(cluster=w746, "type"="Lifetime (scan)") -> (w744:T11)
                        n3998 = call "2pparameters.vi"("Params in"=w744, "command"="set") -> ()  [unwired: 1 out]
                      }
                      frame "Lifetime (contour)" {
                        n3999 = local read "Vy-min draw"() -> (w756:dbl)
                        n4000 = local read "Vy-max draw"() -> (w755:dbl)
                        n4001 = local read "Vx-min draw"() -> (w758:dbl)
                        n4002 = local read "Vx-max draw"() -> (w757:dbl)
                        n4003 = local read "xpixels ref"() -> (w754:i32)
                        n4004 = local read "ypixels ref"() -> (w753:i32)
                        n4005 = local read "ROI Type"() -> (w752:u16)
                        n4006 = local read "srateAODOtt"() -> (w763:dbl)
                        n4007 = local read "# of frames"() -> (w768:i32)
                        n4008 = local read "refreshtime"() -> (w760:dbl)
                        n4009 = local read "Pel"() -> (w751:dbl)
                        n4010 = local read "bin"() -> (w766:dbl)
                        n4011 = local read "Override AI buffer"() -> (w749:bool)
                        n4012 = local read "finite samples"() -> (w775:bool)
                        n4013 = local read "srateAODOtt"() -> (w762:dbl)
                        n4014 = local read "srateAODOtt"() -> (w769:dbl)
                        n4015 = local read "continuous"() -> (w774:bool)
                        n4016 = local read "Angle ref"() -> (w759:dbl)
                        n4017 = local read "wavdet"() -> (w776:bool)
                        n4018 = local read "Vx-ref"() -> (w771:dbl)
                        n4019 = local read "Vy-ref"() -> (w773:dbl)
                        n4020 = local read "avpp"() -> (w772:i32)
                        n4021 = call "tt_timeandsamples.vi"("bin"=w766, "refreshtime"=w760, "srateAODOtt"=w763, "tot#ofsamples"=w768) -> ("refreshrate"=w764:dbl, "refreshbuffer"=w765:i32, "timetracecycles"=w770:i32)  [unwired: 5 in]
                        n4022 = local read "bin"() -> (w767:dbl)
                        n4023 = call "2pparameters.vi"("command"="get") -> ("params out"=w779:T11)  [unwired: 1 in]
                        n4024 = Bundle By Name(cluster=w779, "Drawing Mode"=w752, "measpoints"=w768, "tt_cycles"=w770, "refreshbuffer"=w765, "refreshrate"=w764, "Vx-ref"=w771, "Vy-ref"=w773, "srate"=w762, "finite"=w775, "cont"=w774, "wavdet"=w776, "avpp"=w772, "srateAODO"=w769, "bufferAI"=w765, "bin"=w767, "Angle Img"=w759, "Vxminref"=w758, "Vxmaxref"=w757, "Vyminref"=w756, "Vymaxref"=w755, "Xpixels Img"=w754, "Ypixels Img"=w753, "Pel"=w751, "Vz-reset"=0.0, "AIoverride"=w749, "type"="Lifetime (contour)") -> (w777:T11)
                        n4025 = Reciprocal(x=w764) -> (1/x=w761:dbl)
                        n4026 = local write "refreshtime"(w761) -> ()
                        n4027 = call "2pparameters.vi"("Params in"=w777, "command"="set") -> ()  [unwired: 1 out]
                      }
                      frame "X-Y-Z-t movie" {
                      }
                      frame "linescan" {
                      }
                      frame "Timetrace" {
                        n4028 = local read "Vy-min draw"() -> (w789:dbl)
                        n4029 = local read "Vy-max draw"() -> (w788:dbl)
                        n4030 = local read "Vx-min draw"() -> (w791:dbl)
                        n4031 = local read "Vx-max draw"() -> (w790:dbl)
                        n4032 = local read "xpixels ref"() -> (w787:i32)
                        n4033 = local read "ypixels ref"() -> (w786:i32)
                        n4034 = local read "ROI Type"() -> (w785:u16)
                        n4035 = local read "srateAODOtt"() -> (w796:dbl)
                        n4036 = local read "# of frames"() -> (w801:i32)
                        n4037 = local read "refreshtime"() -> (w793:dbl)
                        n4038 = local read "Pel"() -> (w784:dbl)
                        n4039 = local read "bin"() -> (w799:dbl)
                        n4040 = local read "Override AI buffer"() -> (w782:bool)
                        n4041 = local read "finite samples"() -> (w808:bool)
                        n4042 = local read "srateAODOtt"() -> (w795:dbl)
                        n4043 = local read "srateAODOtt"() -> (w802:dbl)
                        n4044 = local read "continuous"() -> (w807:bool)
                        n4045 = local read "Angle ref"() -> (w792:dbl)
                        n4046 = local read "wavdet"() -> (w809:bool)
                        n4047 = local read "Vx-ref"() -> (w804:dbl)
                        n4048 = local read "Vy-ref"() -> (w806:dbl)
                        n4049 = local read "avpp"() -> (w805:i32)
                        n4050 = call "tt_timeandsamples.vi"("bin"=w799, "refreshtime"=w793, "srateAODOtt"=w796, "tot#ofsamples"=w801) -> ("refreshrate"=w797:dbl, "refreshbuffer"=w798:i32, "timetracecycles"=w803:i32)  [unwired: 5 in]
                        n4051 = local read "bin"() -> (w800:dbl)
                        n4052 = call "2pparameters.vi"("command"="get") -> ("params out"=w812:T11)  [unwired: 1 in]
                        n4053 = Bundle By Name(cluster=w812, "Drawing Mode"=w785, "measpoints"=w801, "tt_cycles"=w803, "refreshbuffer"=w798, "refreshrate"=w797, "Vx-ref"=w804, "Vy-ref"=w806, "srate"=w795, "finite"=w808, "cont"=w807, "wavdet"=w809, "avpp"=w805, "srateAODO"=w802, "bufferAI"=w798, "bin"=w800, "Angle Img"=w792, "Vxminref"=w791, "Vxmaxref"=w790, "Vyminref"=w789, "Vymaxref"=w788, "Xpixels Img"=w787, "Ypixels Img"=w786, "Pel"=w784, "Vz-reset"=0.0, "AIoverride"=w782, "type"="Timetrace") -> (w810:T11)
                        n4054 = Reciprocal(x=w797) -> (1/x=w794:dbl)
                        n4055 = local write "refreshtime"(w794) -> ()
                        n4056 = call "2pparameters.vi"("Params in"=w810, "command"="set") -> ()  [unwired: 1 out]
                      }
                      frame "Lifetime (point)" {
                      }
                    }
                  }
                  frame #1 {
                    w815 = FALSE ("wavdet")
                    n4057 = call "2pparameters.vi"("command"="get") -> ("params out"=w819:T11)  [unwired: 1 in]
                    n4058 = Bundle By Name(cluster=w819, "finite"=w815, "cont"=w815, "wavdet"=TRUE) -> (w816:T11)
                    n4059 = call "2pparameters.vi"("Params in"=w816, "command"="set") -> ()  [unwired: 1 out]
                  }
                  frame #2 {
                    n4060 = local read "DO channels"() -> (w827:u16)
                    n4061 = call "2pparameters.vi"("command"="get") -> ("params out"=w825:T11)  [unwired: 1 in]
                    n4062 = in-place {
                      in-place-border: w827 -> [w832]
                      in-place-border: [w829] -> w822
                      in-place-border: [w828] -> w821
                      n4063 = in-place-cluster #52(w825) -> ("aDO"=w831:u32[])
                      n4064 = call "remove channel from active arrayv2.vi"("line array in"=w831, "line to remove"=w832) -> ("line array out"=w830:u32[], "removal"=w829:bool, "index"=w828:i32)
                      n4065 = in-place-cluster #52("aDO"=w830) -> (w823:T11)
                    }
                    n4066 = local write "remDO"(w822) -> ()
                    n4067 = call "2pparameters.vi"("Params in"=w823, "command"="set") -> ()  [unwired: 1 out]
                  }
                  frame #3 {
                    n4068 = local read "remDO"() -> (w833:bool)
                    n4069 = case shown="True" w833 {
                      frame False {
                      }
                      frame True {
                        n4070 = call "Used AO lines.vi"() -> ("used AO names"=w837:string[], "used AO lines"=w839:tag[])  [unwired: 2 in]
                        n4071 = local write "Analog Used Lines"(w839) -> ()
                        n4072 = local write "Analog Used Names"(w837) -> ()
                        n4073 = call "Used DO lines.vi"() -> ("used DO names"=w835:string[], "used DO lines"=w834:tag[])  [unwired: 2 in]
                        n4074 = control-ref of="Analog Lines Plot"() -> (w838:refnum<vi>)
                        n4075 = control-ref of="Digital Lines Plot"() -> (w836:refnum<vi>)
                        n4076 = local write "Digital Used Lines"(w834) -> ()
                        n4077 = local write "Digital Used Names"(w835) -> ()
                        n4078 = call "prepAOWaveplot.vi"("WaveformGraph in"=w838, "Analog Used Names"=w837) -> ()  [unwired: 1 in]
                        n4079 = call "prepDOWaveplot.vi"("DigitalGraph in"=w836, "used DO names"=w835) -> ()  [unwired: 1 in]
                      }
                    }
                  }
                  frame #4 {
                    n4080 = local read "remDO"() -> (w841:bool)
                    n4081 = case shown="True" w841 {
                      tunnel: w840 -> [_ w842]
                      frame False {
                      }
                      frame True {
                        n4082 = call "waveformparamsv2.vi"("command"="rem DO", "index"=w842) -> ()  [unwired: 3 in, 3 out]
                      }
                    }
                  }
                  frame #5 {
                    n4083 = local read "Meastab"() -> (w847:enum32{"X-Y Image", "Linescan", "Timetrace"})
                    n4084 = property on="refwf" class="Ring (strict)"() -> ("RingText.Text"=w854:string)  [unwired: 2 in, 2 out]
                    n4085 = call "waveformsDObuffer.vi"("command"="get") -> ("DO wf out"=w853:digitalwaveform[])  [unwired: 1 in]
                    n4086 = case shown="\"Timetrace\"" w847 {
                      tunnel: [w863 w864] -> w846
                      frame "X-Y Image", Default {
                        n4087 = local read "Sampling rate"() -> (w863:dbl)
                      }
                      frame "Timetrace" {
                        n4088 = local read "srateAODOtt"() -> (w864:dbl)
                      }
                    }
                    n4089 = call "waveformsAObuffer.vi"("command"="get") -> ("AO wf out"=w862:waveform(dbl)[])  [unwired: 1 in]
                    n4090 = Delete From Array(array=w853, length=1, index=w851) -> (array with subset deleted=w850:digitalwaveform[])  [unwired: 1 out]
                    n4091 = call "correctwaveformsizetemp.vi"("new sampling frequency (Hz)"=w846, "start"=FALSE, "reference waveforms to"=w854, "Analog waveforms in"=w862, "stop"=FALSE, "Digital waveforms in"=w850) -> ("analog wf out"=w857:waveform(dbl)[], "Digital wf out"=w855:digitalwaveform[], "measpoints"=w848:i32)
                    n4092 = local read "wavdet"() -> (w849:bool)
                    n4093 = call "waveformsAObuffer.vi"("AO wf in"=w857, "command"="set") -> ()  [unwired: 1 out]
                    n4094 = call "waveformsDObuffer.vi"("DO wf in"=w855, "command"="set") -> ()  [unwired: 1 out]
                    n4095 = local write "Analog Lines Plot"(w857) -> ()
                    n4096 = local write "Digital Lines Plot"(w855) -> ()
                    n4097 = call "GetNumCamFramesv2.vi"("Digital Waveform Graph"=w855) -> ("Numeric"=w856:i32)  [unwired: 10 in]
                    n4098 = case shown="True" w849 {
                      tunnel: w848 -> [_ w865]
                      frame False {
                      }
                      frame True {
                        n4099 = local write "# of frames"(w865) -> ()
                      }
                    }
                    n4100 = local write "Total Camera Frames"(w856) -> ()
                  }
                  frame #6 {
                    w866 = FALSE ("addAO")
                    n4101 = local read "finite samples"() -> (w867:bool)
                    n4102 = local read "continuous"() -> (w868:bool)
                    n4103 = local read "wavdet"() -> (w869:bool)
                    n4104 = local write "remDO"(w866) -> ()
                    n4105 = call "2pparameters.vi"("command"="get") -> ("params out"=w872:T11)  [unwired: 1 in]
                    n4106 = Bundle By Name(cluster=w872, "finite"=w867, "cont"=w868, "wavdet"=w869) -> (w870:T11)
                    n4107 = property on="Rem DO wave" class="Bool (strict)"("Val(Sgnl)"=w866) -> ()  [unwired: 2 in, 2 out]
                    n4108 = call "2pparameters.vi"("Params in"=w870, "command"="set") -> ()  [unwired: 1 out]
                  }
                }
              }
            }
          }
          event "Digital phase (s)", "Digital DC (%)", "Digital Freq (Hz)", "Digital padding value", "Digital time offset (s)": Value Change {
            n4109 = event-data() -> ()  [unwired: 1 in, 6 out]
            n4110 = stacked-sequence {
              seq-local: [_ _ w980 _ _] -> [_ _ _ w997 _]
              seq-local: [_ _ w979 _ _] -> [_ _ _ w996 _]
              frame #0 {
                n4111 = local read "Measurement"() -> (w874:T4)
                n4112 = case shown="\"X-Y-t movie\", Default" w874 {
                  frame "X-Y-t movie", Default {
                    n4113 = local read "avpp"() -> (w895:i32)
                    n4114 = local read "Angle ref"() -> (w894:dbl)
                    n4115 = local read "ROI Type"() -> (w893:u16)
                    n4116 = local read "xpixels ref"() -> (w890:i32)
                    n4117 = local read "Vx-min ref"() -> (w889:dbl)
                    n4118 = local read "Vx-max ref"() -> (w888:dbl)
                    n4119 = local read "ypixels ref"() -> (w886:i32)
                    n4120 = local read "Vy-min ref"() -> (w887:dbl)
                    n4121 = local read "Vy-max ref"() -> (w883:dbl)
                    n4122 = local read "Sampling rate"() -> (w877:dbl)
                    n4123 = local read "finite samples"() -> (w878:bool)
                    n4124 = local read "continuous"() -> (w881:bool)
                    n4125 = local read "wavdet"() -> (w882:bool)
                    n4126 = local read "# of frames"() -> (w880:i32)
                    n4127 = local read "maxbufferAI"() -> (w879:i32)
                    n4128 = local read "Override AI buffer"() -> (w875:bool)
                    n4129 = call "2pparameters.vi"("command"="get") -> ("params out"=w892:T11)  [unwired: 1 in]
                    n4130 = Bundle By Name(cluster=w892, "type"="X-Y-t movie", "avpp"=w895, "Angle Img"=w894, "Xpixels Img"=w890, "Vx-min Img"=w889, "VX-max Img"=w888, "Ypixels Img"=w886, "Vy-min Img"=w887, "Vy-max Img"=w883, "srate"=w877, "srate Img"=w877, "finite"=w878, "cont"=w881, "wavdet"=w882, "measpoints"=w880, "maxbufferAI"=w879, "Drawing Mode"=w893, "Vz-reset"=0.0, "AIoverride"=w875) -> (w884:T11)
                    n4131 = call "2pparameters.vi"("Params in"=w884, "command"="set") -> ()  [unwired: 1 out]
                  }
                  frame "X-Y-Z stack" {
                    n4132 = call "2pparameters.vi"("command"="get") -> ("params out"=w899:T11)  [unwired: 1 in]
                    n4133 = Bundle By Name(cluster=w899, "type"="X-Y-Z stack") -> (w897:T11)
                    n4134 = call "2pparameters.vi"("Params in"=w897, "command"="set") -> ()  [unwired: 1 out]
                  }
                  frame "Lifetime (scan)" {
                    n4135 = call "2pparameters.vi"("command"="get") -> ("params out"=w904:T11)  [unwired: 1 in]
                    n4136 = Bundle By Name(cluster=w904, "type"="Lifetime (scan)") -> (w902:T11)
                    n4137 = call "2pparameters.vi"("Params in"=w902, "command"="set") -> ()  [unwired: 1 out]
                  }
                  frame "Lifetime (contour)" {
                    n4138 = local read "Vy-min draw"() -> (w914:dbl)
                    n4139 = local read "Vy-max draw"() -> (w913:dbl)
                    n4140 = local read "Vx-min draw"() -> (w916:dbl)
                    n4141 = local read "Vx-max draw"() -> (w915:dbl)
                    n4142 = local read "xpixels ref"() -> (w912:i32)
                    n4143 = local read "ypixels ref"() -> (w911:i32)
                    n4144 = local read "ROI Type"() -> (w910:u16)
                    n4145 = local read "srateAODOtt"() -> (w921:dbl)
                    n4146 = local read "# of frames"() -> (w926:i32)
                    n4147 = local read "refreshtime"() -> (w918:dbl)
                    n4148 = local read "Pel"() -> (w909:dbl)
                    n4149 = local read "bin"() -> (w924:dbl)
                    n4150 = local read "Override AI buffer"() -> (w907:bool)
                    n4151 = local read "finite samples"() -> (w933:bool)
                    n4152 = local read "srateAODOtt"() -> (w920:dbl)
                    n4153 = local read "srateAODOtt"() -> (w927:dbl)
                    n4154 = local read "continuous"() -> (w932:bool)
                    n4155 = local read "Angle ref"() -> (w917:dbl)
                    n4156 = local read "wavdet"() -> (w934:bool)
                    n4157 = local read "Vx-ref"() -> (w929:dbl)
                    n4158 = local read "Vy-ref"() -> (w931:dbl)
                    n4159 = local read "avpp"() -> (w930:i32)
                    n4160 = call "tt_timeandsamples.vi"("bin"=w924, "refreshtime"=w918, "srateAODOtt"=w921, "tot#ofsamples"=w926) -> ("refreshrate"=w922:dbl, "refreshbuffer"=w923:i32, "timetracecycles"=w928:i32)  [unwired: 5 in]
                    n4161 = local read "bin"() -> (w925:dbl)
                    n4162 = call "2pparameters.vi"("command"="get") -> ("params out"=w937:T11)  [unwired: 1 in]
                    n4163 = Bundle By Name(cluster=w937, "Drawing Mode"=w910, "measpoints"=w926, "tt_cycles"=w928, "refreshbuffer"=w923, "refreshrate"=w922, "Vx-ref"=w929, "Vy-ref"=w931, "srate"=w920, "finite"=w933, "cont"=w932, "wavdet"=w934, "avpp"=w930, "srateAODO"=w927, "bufferAI"=w923, "bin"=w925, "Angle Img"=w917, "Vxminref"=w916, "Vxmaxref"=w915, "Vyminref"=w914, "Vymaxref"=w913, "Xpixels Img"=w912, "Ypixels Img"=w911, "Pel"=w909, "Vz-reset"=0.0, "AIoverride"=w907, "type"="Lifetime (contour)") -> (w935:T11)
                    n4164 = Reciprocal(x=w922) -> (1/x=w919:dbl)
                    n4165 = local write "refreshtime"(w919) -> ()
                    n4166 = call "2pparameters.vi"("Params in"=w935, "command"="set") -> ()  [unwired: 1 out]
                  }
                  frame "X-Y-Z-t movie" {
                  }
                  frame "linescan" {
                  }
                  frame "Timetrace" {
                    n4167 = local read "Vy-min draw"() -> (w947:dbl)
                    n4168 = local read "Vy-max draw"() -> (w946:dbl)
                    n4169 = local read "Vx-min draw"() -> (w949:dbl)
                    n4170 = local read "Vx-max draw"() -> (w948:dbl)
                    n4171 = local read "xpixels ref"() -> (w945:i32)
                    n4172 = local read "ypixels ref"() -> (w944:i32)
                    n4173 = local read "ROI Type"() -> (w943:u16)
                    n4174 = local read "srateAODOtt"() -> (w954:dbl)
                    n4175 = local read "# of frames"() -> (w959:i32)
                    n4176 = local read "refreshtime"() -> (w951:dbl)
                    n4177 = local read "Pel"() -> (w942:dbl)
                    n4178 = local read "bin"() -> (w957:dbl)
                    n4179 = local read "Override AI buffer"() -> (w940:bool)
                    n4180 = local read "finite samples"() -> (w966:bool)
                    n4181 = local read "srateAODOtt"() -> (w953:dbl)
                    n4182 = local read "srateAODOtt"() -> (w960:dbl)
                    n4183 = local read "continuous"() -> (w965:bool)
                    n4184 = local read "Angle ref"() -> (w950:dbl)
                    n4185 = local read "wavdet"() -> (w967:bool)
                    n4186 = local read "Vx-ref"() -> (w962:dbl)
                    n4187 = local read "Vy-ref"() -> (w964:dbl)
                    n4188 = local read "avpp"() -> (w963:i32)
